vi "Operator message box key exit.vi"(8 "error in (no error)":errorcluster, 10 "Font:Size":u32=18, 11 "Text message":string) -> (0 "error out":errorcluster)   [LabVIEW 2013]
panel:
  out "String":string
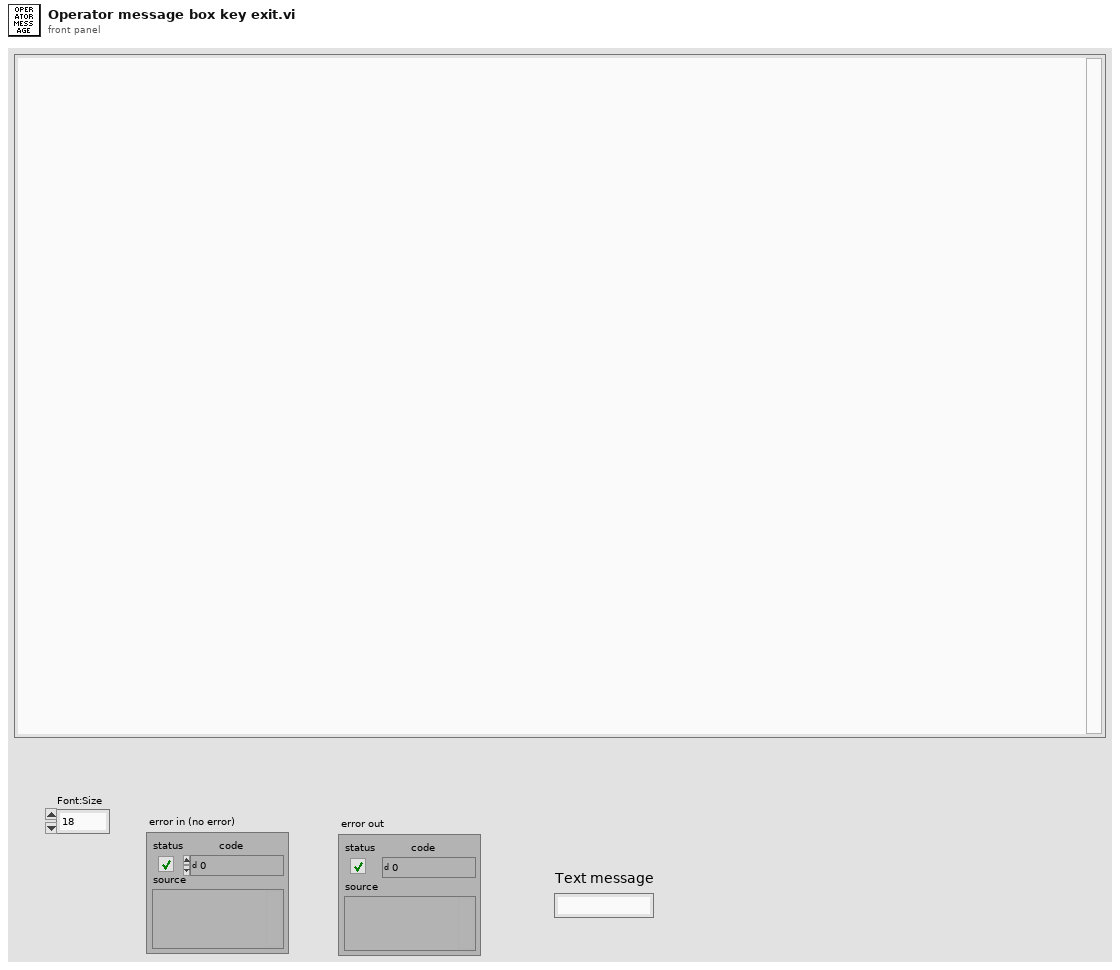
[diagram p1: front panel]
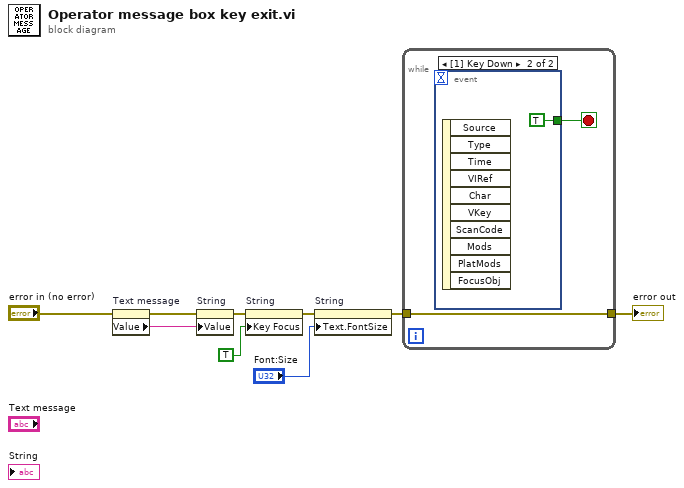
[diagram p0: block diagram]
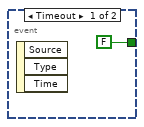
[diagram p2: hidden frame]
diagram:
  n1 = property on="Text message" class="Str"(error in="error in (no error)") -> (error out=w3:errorcluster, "Value"=w4:string)  [unwired: 1 in, 1 out]
  n2 = property on="String" class="Str"(error in=w3, "Value"=w4) -> (error out=w1:errorcluster)  [unwired: 1 in, 1 out]
  n3 = property on="String" class="Str"(error in=w1, "Key Focus"=TRUE) -> (error out=w7:errorcluster)  [unwired: 1 in, 1 out]
  n4 = property on="String" class="Str"(error in=w7, "Text.FontSize"="Font:Size") -> (error out=w5:errorcluster)  [unwired: 1 in, 1 out]
  n5 = while {
    tunnel: [w10] -> w6
    tunnel: w5 -> [w10]
    stop <- w11 stop-if-true
    n6 = event shown="[1] Key Down" {
      selector: _ -> [_ _]
      dyn-events: _ -> [_ _]
      timeout: _ -> [_ _]
      tunnel: [FALSE ("stop? (T)") TRUE ("stop? (T)")] -> w11
      event Timeout {
        n7 = event-data() -> ()  [unwired: 1 in, 3 out]
      }
      event Key Down {
        n8 = event-data() -> ()  [unwired: 1 in, 10 out]
      }
    }
  }
  "error out" <- w6
